vi "Source Voltage.vi"(7 "Channel Lists":string[](array[string]), 8 "error in (no error)":errorcluster, 10 "voltage level":dbl format="%_6p", 11 "Instrument Sessions In":refnum<k15>[](array[refnum])) -> (0 "error out":errorcluster, 1 "current measurements":dbl[][](array[numeric]), 2 "voltage measurements":dbl[][](array[numeric]), 3 "Instrument Sessions Out":refnum<k15>[](array[refnum]))   [LabVIEW 2013]
uses:
  <instrlib>/niDCPower/nidcpower.llb/niDCPower Wait For Event - Event.ctl
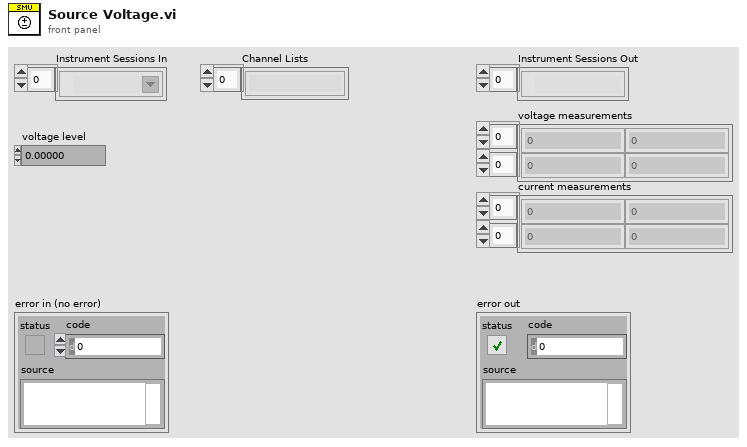
[diagram p1: front panel]
types:
  T1 = typedef "niDCPower Wait For Event - Event.ctl" = i32
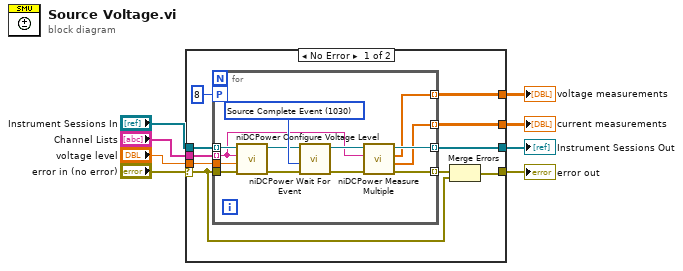
[diagram p0: block diagram]
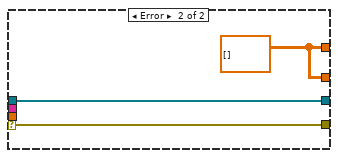
[diagram p2: hidden frame]
diagram:
  n1 = case shown="No Error" "error in (no error)" {
    selector: "error in (no error)" -> [w10 w33]
    tunnel: [w17 w33] -> w8
    tunnel: "Instrument Sessions In" -> [w16 w34]
    tunnel: "Channel Lists" -> [w15 _]
    tunnel: [w14 w34] -> w5
    tunnel: "voltage level" -> [w13 _]
    tunnel: [w12 w32] -> w2
    tunnel: [w11 w32] -> w1
    frame No Error {
      n2 = for {
        tunnel: w16 -> [w31] mode=indexing
        tunnel: w15 -> [w23] mode=indexing
        tunnel: [w22] -> w14 mode=indexing
        tunnel: [w21] -> w18 mode=indexing
        tunnel: w13 -> [w30]
        tunnel: w10 -> [w29]
        tunnel: [w20] -> w12 mode=indexing
        tunnel: [w19] -> w11 mode=indexing
        workers-P: 8 -> [_]
        w27 = T1 1030 items=["Source Complete Event"=1030, "Measure Complete Event"=1031, "Sequence Iteration Complete Event"=1032, "Sequence Engine Done Event"=1033, "Pulse Complete Event"=1051, "Ready For Pulse Trigger Event"=1052] ("event")
        n3 = call <instrlib>:"niDCPower Configure Voltage Level.vi"("error in (no error)"=w29, "voltage level"=w30, "channel name"=w23, "instrument handle"=w31) -> ("error out"=w28:errorcluster, "instrument handle out"=w26:refnum<k15>)  [unwired: 6 in]
        n4 = call <instrlib>:"niDCPower Wait For Event.vi"("error in (no error)"=w28, "event"=w27, "instrument handle"=w26) -> ("error out"=w25:errorcluster, "instrument handle out"=w24:refnum<k15>)  [unwired: 7 in]
        n5 = call <instrlib>:"niDCPower Measure Multiple.vi"("error in (no error)"=w25, "channel name"=w23, "instrument handle"=w24) -> ("error out"=w21:errorcluster, "current measurements"=w19:dbl[], "voltage measurements"=w20:dbl[], "instrument handle out"=w22:refnum<k15>)  [unwired: 5 in]
      }
      n6 = Merge Errors(w18, w10) -> (w17:errorcluster)
    }
    frame Error {
      w32 = dbl[][] [] ("voltage measurements")
    }
  }
  "Instrument Sessions Out" <- w5
  "error out" <- w8
  "voltage measurements" <- w2
  "current measurements" <- w1
